vi "GetOutputType.vi"(7 "DLL path":path, 8 "error in (no error)":errorcluster, 10 "outputIndex":i32, 11 "session id in":i32) -> (0 "error out":errorcluster, 2 "OutputTypeIndex":i32, 3 "session id out":i32)   [LabVIEW 2017, in "ONNX Class Library.lvlib"]
doc: "/**\n * @brief Получить код типа данных входного тензора\n * \n * Возвращает числовой код типа элементов тензора согласно спецификации ONNX.\n * Используйте таблицу констант в начале этого файла для расшифровки.\n * \n * @param sessionId [IN] ID сессии\n * @param inputIndex [IN] Индекс входа (0-based)\n * \n * @return int32: Код типа данных (1=FLOAT32, 2=FLOAT64, 5=INT32, 6=INT64, ...)\n * @return int32: -1 если сессия не найдена или индекс неверен\n * \n * @see GetInputTypeString для получения читаемого имени типа\n */\nint GetInputType(int sessionId, int inputIndex);"
uses:
  ONNX Class Library.lvlib
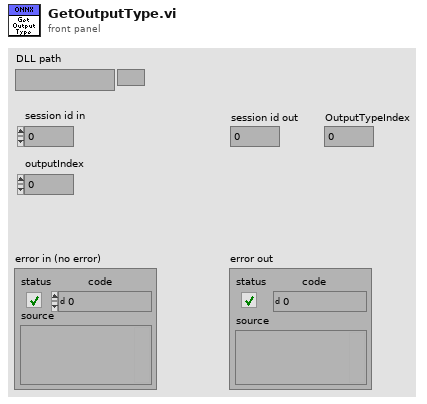
[diagram p1: front panel]
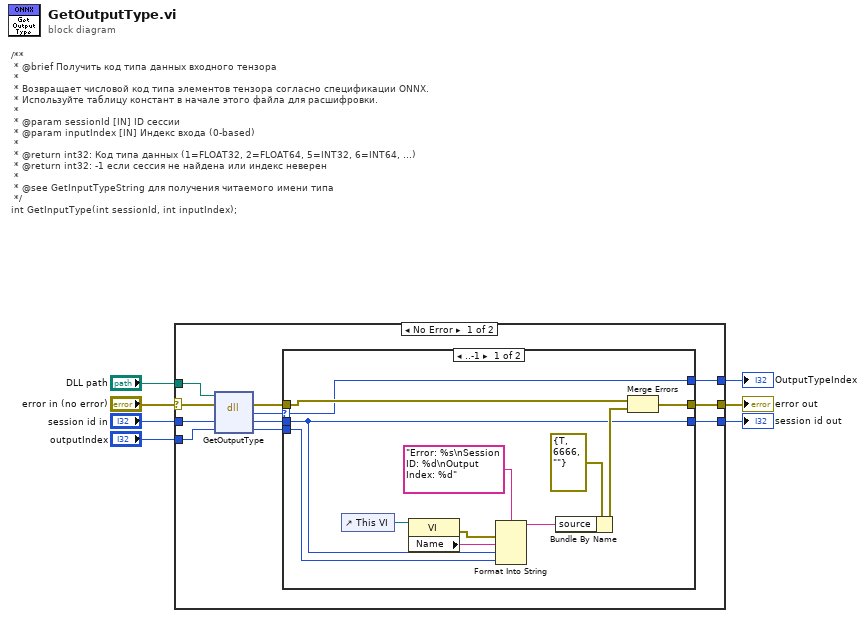
[diagram p0: block diagram]
diagram:
  # "/**\n * @brief Получить код типа данных входного тензора\n * \n * Возвращает числовой код типа элементов тензора согласно спецификации ONNX.\n * Используйте таблицу констант в начале этого файла для расшифровки.\n * \n * @param sessionId [IN] ID сессии\n * @param inputIndex [IN] Индекс входа (0-based)\n * \n * @return int32: Код типа данных (1=FLOAT32, 2=FLOAT64, 5=INT32, 6=INT64, ...)\n * @return int32: -1 если сессия не найдена или индекс неверен\n * \n * @see GetInputTypeString для получения читаемого имени типа\n */\nint GetInputType(int sessionId, int inputIndex);"
  n1 = case shown="No Error" "error in (no error)" {
    selector: "error in (no error)" -> [w9 w35]
    tunnel: "outputIndex" -> [w18 _]
    tunnel: "session id in" -> [w17 w34]
    tunnel: [w12 w35] -> w5
    tunnel: [w11 w34] -> w4
    tunnel: [w10 _] -> w3
    tunnel: "DLL path" -> [w8 _]
    frame No Error {
      n2 = dll-call lib="home/ivan/LabVIEWData/ONNX/Test/libonnx_wrapper/unix64/libonnx_wrapper.so" fn="GetOutputType"(path in=w8, error in=w9, "sessionId"=w17, "outputIndex"=w18) -> (error out=w16:errorcluster, "OutputTypeIndex"=w15:i32, "sessionId"=w14:i32, "outputIndex"=w13:i32)  [unwired: 1 in, 1 out]
      n3 = case shown="..-1" w15 {
        selector: w15 -> [w19 w31]
        tunnel: w16 -> [w21 w33]
        tunnel: [w22 w33] -> w12
        tunnel: w14 -> [w23 w32]
        tunnel: [w23 w32] -> w11
        tunnel: w13 -> [w20 _]
        tunnel: [w19 w31] -> w10
        frame ..-1 {
          n4 = control-ref of="This VI"() -> (w27:refnum<vi>)
          n5 = property class="VI"(reference=w27) -> (error out=w24:errorcluster, "Name"=w26:string)  [unwired: 1 in, 1 out]
          n6 = Format Into String(format string="Error: %s\nSession ID: %d\nOutput Index: %d", error in=w24, w26, w23, w20) -> (resulting string=w28:string)  [unwired: 1 in, 1 out]
          n7 = Bundle By Name(cluster=errorcluster {"status"=TRUE, "code"=6666, "source"=""} ("error out"), "source"=w28) -> (w29:errorcluster)
          n8 = Merge Errors(w21, w29) -> (w22:errorcluster)
        }
        frame 0.. {
        }
      }
    }
    frame Error {
    }
  }
  "error out" <- w5
  "session id out" <- w4
  "OutputTypeIndex" <- w3
